vi "Write configuration.vi"(8 "error in (no error)":errorcluster, 11 "Template in":refnum<class "BMC.lvclass">) -> (0 "error out":errorcluster, 3 "Template out":refnum<class "BMC.lvclass">)   [LabVIEW 2012]
doc: "Writes the configuration cluster into the configuration file. Configuration file is XML-based. It's name is <component ID>.xml"
uses:
  <vilib>/Distrio/Murmex/Murmex/Murmex.lvclass
  BMC.lvclass
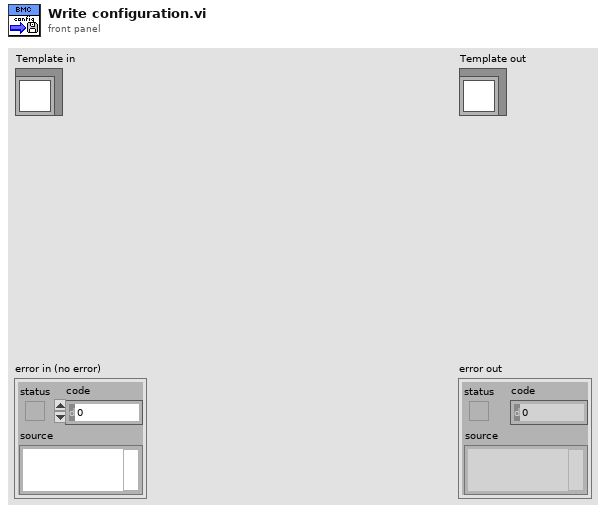
[diagram p1: front panel]
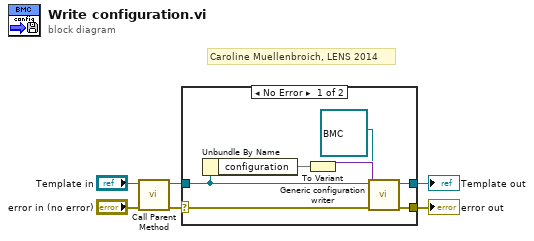
[diagram p0: block diagram]
diagram:
  # "Caroline Muellenbroich, LENS 2014"
  n1 = call-parent "Call Parent Method"("error in (no error)"="error in (no error)", "Murmex in"="Template in") -> ("error out"=w4:errorcluster, "Murmex out"=w2:refnum<class "BMC.lvclass">)  [unwired: 8 in]
  n2 = case shown="No Error" w4 {
    selector: w4 -> [w12 w15]
    tunnel: [w11 w15] -> w3
    tunnel: [w8 w14] -> w1
    tunnel: w2 -> [w9 w14]
    frame No Error {
      n3 = Unbundle By Name(w9) -> ("configuration"=w13)
      n4 = To Variant(anything=w13) -> (Variant=w10:variant)
      n5 = call <vilib>:"Generic configuration writer.vi"("error in (no error)"=w12, 9:w10, 10:refnum<class "BMC.lvclass"> refnum ("Template.lvclass"), "Murmex in"=w9) -> ("error out"=w11:errorcluster, "Murmex out"=w8:refnum<class "BMC.lvclass">)  [unwired: 6 in]
    }
    frame Error {
    }
  }
  "error out" <- w3
  "Template out" <- w1
